vi "计算结果-快关试验.vi"(3 "试验模式":string="快关L1", 5 "油动机试验路径":path=path "D:/研究生/课程/油动机项目/实验文件夹/195-15-6203-018/GV1") -> (0 "计算参数 out":T1, 1 "输入参数":T2, 2 "快关实验":cluster{dbl, "Sampling Rate":dbl, dbl[][]}(graph) caption="当前试验模式：快关试验L1")   [LabVIEW 2013]
uses:
  <vilib>/Analysis/3filter.llb/Filter Passband Type.ctl
  <vilib>/Utility/config.llb/Read Key (String).vi
  <vilib>/Analysis/3filter.llb/Butterworth Filter (DBL).vi
  <vilib>/Analysis/NI_AALBase.lvlib
  <vilib>/Utility/config.llb/NI_LVConfig.lvlib
panel:
  in  "计算参数":T1
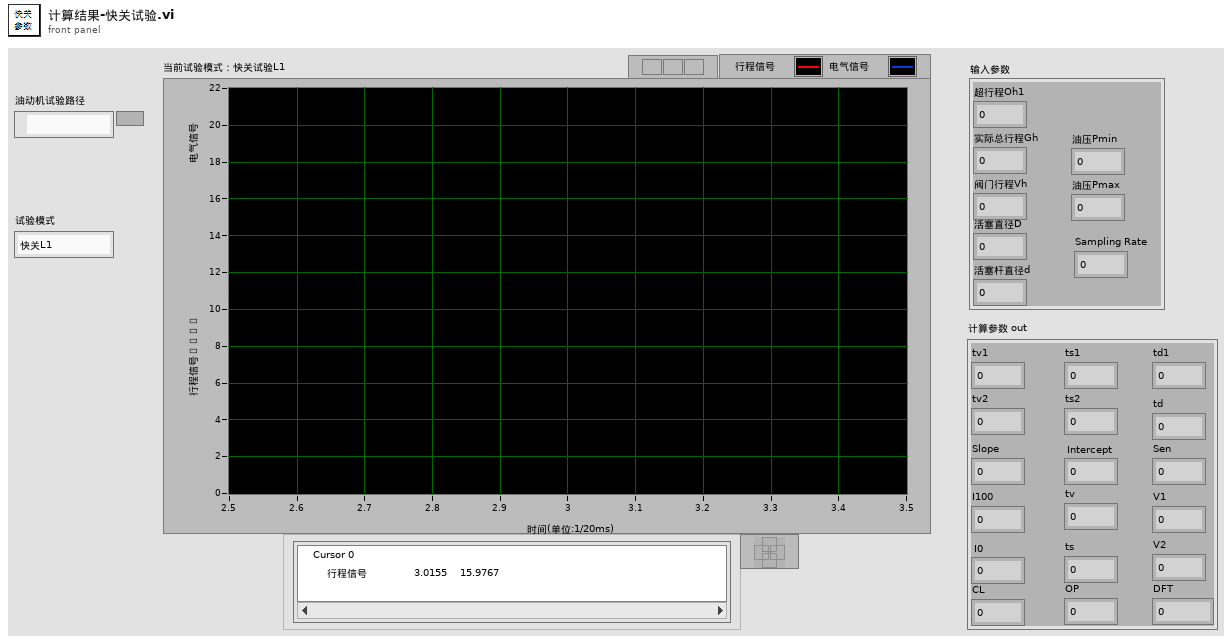
[diagram p1: front panel]
types:
  T1 = cluster{"tv1":dbl, "tv2":dbl, "tv":dbl, "ts1":dbl, "ts2":dbl, "ts":dbl, "td1":dbl, "td":dbl, "Slope":dbl, "Intercept":dbl, "I100":dbl, "I0":dbl, "Sen":dbl, "V1":dbl, "V2":dbl, "CL":dbl, "OP":dbl, "DFT":dbl}
  T2 = cluster{"超行程Oh1":dbl, "实际总行程Gh":dbl, "阀门行程Vh":dbl, "活塞直径D":dbl, "活塞杆直径d":dbl, "油压Pmin":dbl, "油压Pmax":dbl, "Sampling Rate":dbl}
  T3 = typedef "NI_AALBase.lvlib/Filter Passband Type.ctl" = enum32{"Lowpass", "Highpass", "Bandpass", "Bandstop"}
  T4 = enum16{"open", "open or create", "create or replace", "create", "open (read-only)"}
  T5 = typedef "NI_LVConfig.lvlib/Config Data RefNum.ctl" = refnum<k1>
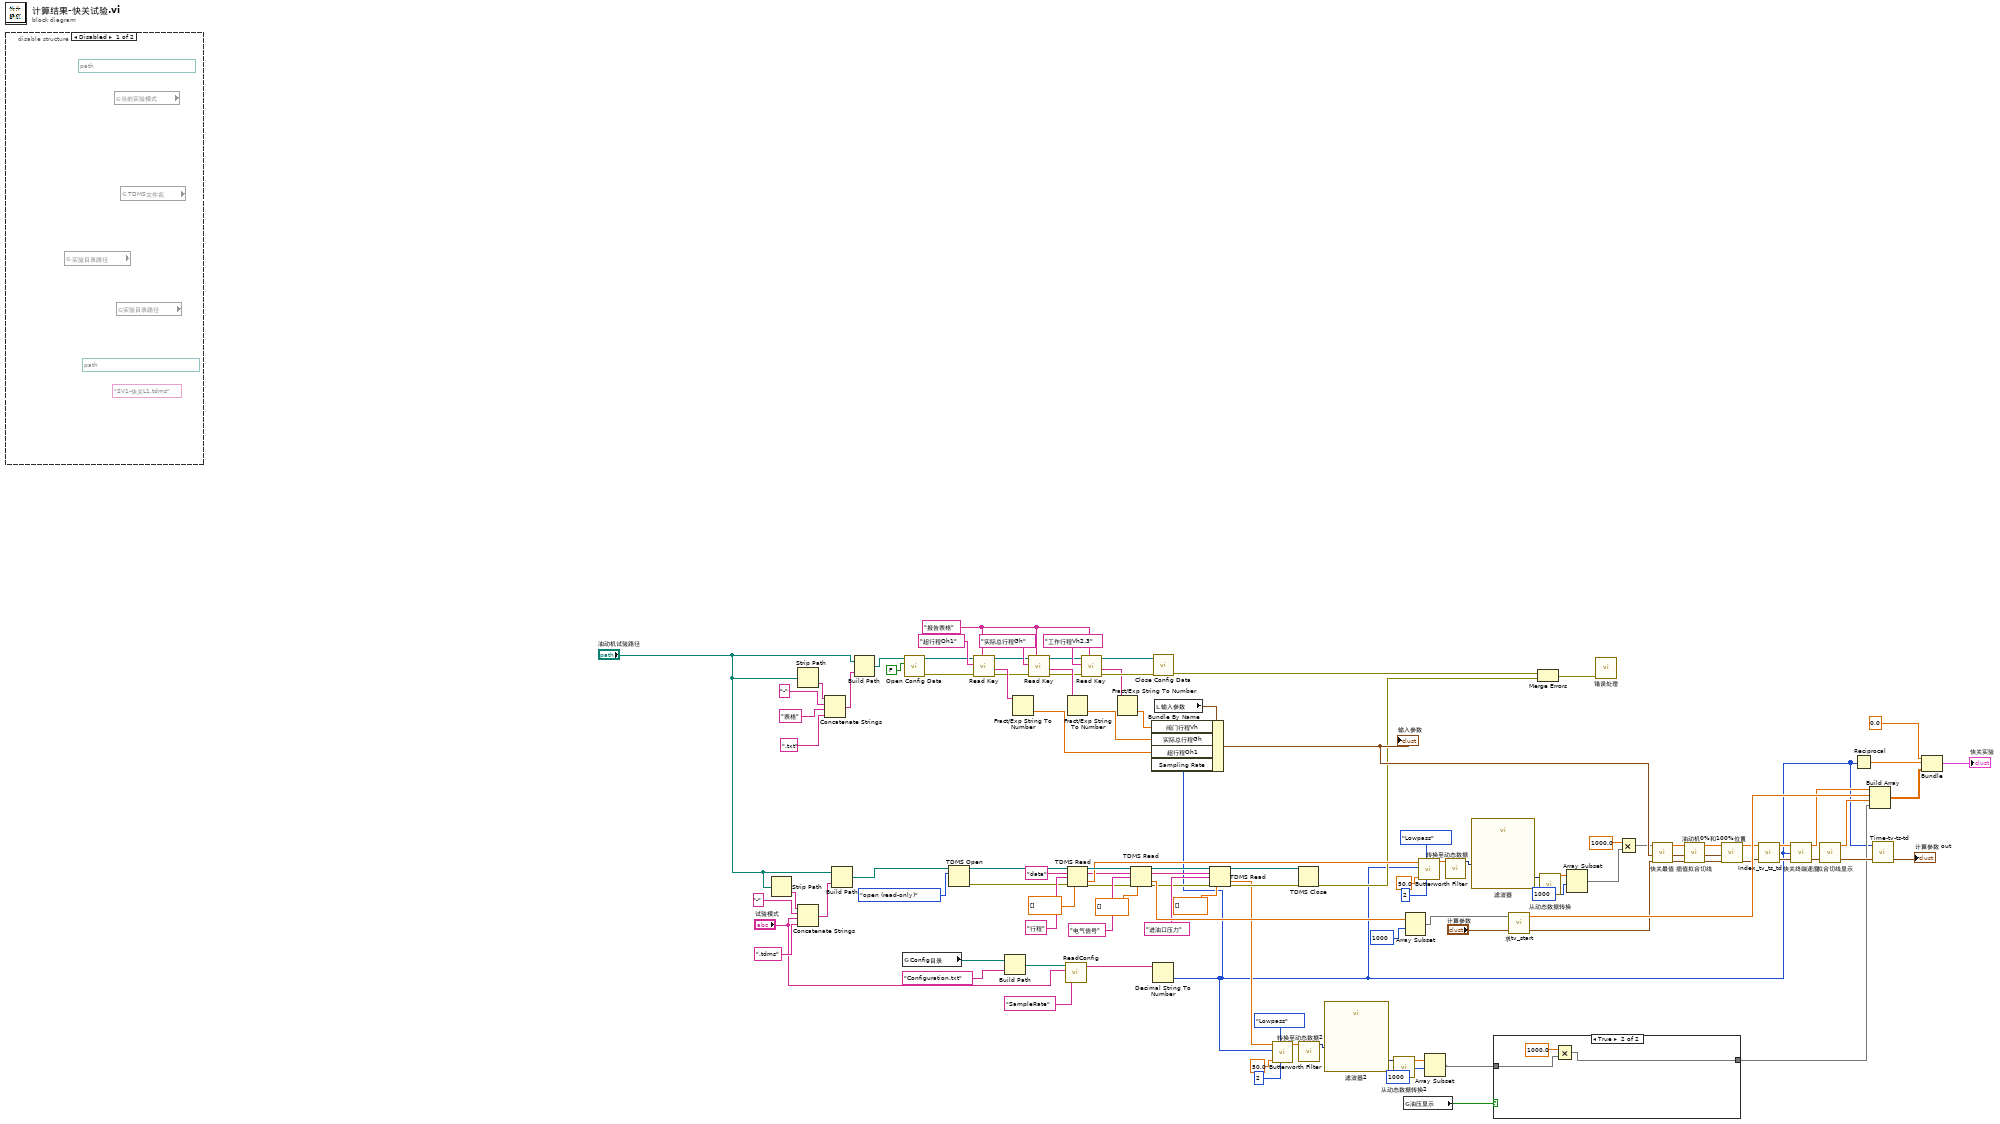
[diagram p0: block diagram]
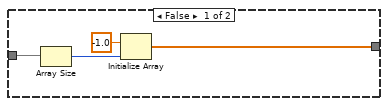
[diagram p2: hidden frame]
diagram:
  w73 = "报告表格" ("section")
  n1 = disable-structure shown="Disabled" {
    frame Disabled {
      (unwired) "SV1-快关L1.tdms"
      (unwired) path "C:/Users/Xiang MU/Desktop/实验文件夹/DR96-03-5/SV1"
      (unwired) path "C:/Users/Xiang MU/Desktop/实验文件夹/DR96-03-5/SV1/SV1-表格.txt"
      n2 = global read "实验目录路径.vi" "实验目录路径"() -> ()  [unwired: 1 out]
      n3 = global read "当前实验模式.vi" "当前实验模式"() -> ()  [unwired: 1 out]
      n4 = global read "实验目录路径.vi" "实验目录路径"() -> ()  [unwired: 1 out]
      n5 = global read "TDMS文件名.vi" "TDMS文件名"() -> ()  [unwired: 1 out]
    }
    frame Enabled {
    }
  }
  n6 = Strip Path(path="油动机试验路径") -> (name=w54:string)  [unwired: 1 out]
  n7 = Strip Path(path="油动机试验路径") -> (name=w49:string)  [unwired: 1 out]
  n8 = Concatenate Strings(w54, "-" ("string"), "试验模式", ".tdms") -> (w53:string)
  n9 = Concatenate Strings(w49, "-" ("string"), "表格" ("string"), ".txt") -> (w45:string)
  n10 = Build Path(base path="油动机试验路径", name or relative path=w53) -> (appended path=w52:path)
  n11 = Build Path(base path="油动机试验路径", name or relative path=w45) -> (appended path=w43:path)
  n12 = global read "Config目录.vi" "Config目录"() -> (w28:path)
  n13 = call <vilib>:"Open Config Data.vi"("create file if necessary (T)"=FALSE, "configuration file path"=w43) -> ("error out"=w58:errorcluster, "refnum"=w57:T5)  [unwired: 7 in, 1 out]
  n14 = TDMS Open(10:T4."open (read-only)" ("operation (0:open)"), 11:w52) -> (0:w26:errorcluster, 3:w55:refnum<k34>)  [unwired: 5 in]
  n15 = call-poly <vilib>:"Read Key.vi"("section"=w73, "error in (no error)"=w58, "key"="超行程Oh1", "refnum"=w57) -> ("error out"=w69:errorcluster, "value"=w76:string, "refnum out"=w70:T5)  [unwired: 4 in, 1 out]
  n16 = Build Path(base path=w28, name or relative path="Configuration.txt") -> (appended path=w27:path)
  n17 = Fract/Exp String To Number(string=w76) -> (number=w90:dbl)  [unwired: 3 in, 1 out]
  n18 = call-poly <vilib>:"Read Key.vi"("section"=w73, "error in (no error)"=w69, "key"="实际总行程Gh" ("default value"), "refnum"=w70) -> ("error out"=w71:errorcluster, "value"=w77:string, "refnum out"=w72:T5)  [unwired: 4 in, 1 out]
  n19 = call "ReadConfig.vi"("Key"="SampleRate", "Section"="试验模式", "Path"=w27) -> ("Value"=w32:string)  [unwired: 1 in, 2 out]
  n20 = Fract/Exp String To Number(string=w77) -> (number=w89:dbl)  [unwired: 3 in, 1 out]
  n21 = TDMS Read(0:w55, 5:"data" ("组名称输入"), 7:"行程" ("组名称输入"), 11:w26, 12:dbl[] []) -> (4:w86:refnum<k34>, 6:w15:string, 10:w81:dbl[], 15:w25:errorcluster)  [unwired: 3 in, 2 out]
  n22 = call-poly <vilib>:"Read Key.vi"("section"=w73, "error in (no error)"=w71, "key"="工作行程Vh2.3", "refnum"=w72) -> ("error out"=w79:errorcluster, "value"=w78:string, "refnum out"=w80:T5)  [unwired: 4 in, 1 out]
  n23 = Fract/Exp String To Number(string=w78) -> (number=w88:dbl)  [unwired: 3 in, 1 out]
  n24 = TDMS Read(0:w86, 5:w15, 7:"电气信号" ("组名称输入"), 11:w25, 12:dbl[] []) -> (4:w19:refnum<k34>, 6:w14:string, 10:w98:dbl[], 15:w16:errorcluster)  [unwired: 3 in, 2 out]
  n25 = Decimal String To Number(string=w32) -> (number=w1:i32)  [unwired: 2 in, 1 out]
  n26 = call <vilib>:"Close Config Data.vi"("error in (no error)"=w79, "refnum"=w80) -> ("error out"=w24:errorcluster)  [unwired: 8 in, 1 out]
  n27 = local read "输入参数"() -> (w91:T2)
  n28 = Bundle By Name(cluster=w91, "阀门行程Vh"=w88, "实际总行程Gh"=w89, "超行程Oh1"=w90, "Sampling Rate"=w1) -> (w103:T2)
  "输入参数" <- w103
  n29 = TDMS Read(0:w19, 5:w14, 7:"进油口压力" ("组名称输入"), 11:w16, 12:dbl[] []) -> (4:w18:refnum<k34>, 10:w2:dbl[], 15:w17:errorcluster)  [unwired: 3 in, 3 out]
  n30 = call-poly <vilib>:"Butterworth Filter.vi"("order"=2, "filter type"=Filter_Passband_Type."Lowpass", "low cutoff freq: fl"=50.0, "sampling freq: fs"=w1, "X"=w2) -> ("Filtered X"=w7:dbl[])  [unwired: 3 in, 1 out]
  n31 = TDMS Close(8:w17, 11:w18) -> (0:w23:errorcluster)  [unwired: 1 out]
  n32 = call "转换至动态数据2"("Array"=w7) -> ("Dynamic Data Type"=w8:dynamicdata)  [unwired: 3 in]
  n33 = call "滤波器2"("Signal"=w8) -> ("Filtered Signal"=w9:dynamicdata)  [unwired: 9 in, 1 out]
  n34 = call "从动态数据转换2"("Dynamic Data Type"=w9) -> ("Array"=w10:dbl[])  [unwired: 3 in]
  n35 = global read "油压显示.vi" "油压显示"() -> (w13:bool)
  n36 = Array Subset(array=w98, index=1000) -> (w100:dbl[])  [unwired: 1 in]
  n37 = call-poly <vilib>:"Butterworth Filter.vi"("order"=2, "filter type"=Filter_Passband_Type."Lowpass", "low cutoff freq: fl"=50.0, "sampling freq: fs"=w1, "X"=w81) -> ("Filtered X"=w65:dbl[])  [unwired: 3 in, 1 out]
  n38 = Array Subset(array=w10, index=1000) -> (w3:dbl[])  [unwired: 1 in]
  n39 = call "转换至动态数据"("Array"=w65) -> ("Dynamic Data Type"=w66:dynamicdata)  [unwired: 3 in]
  n40 = call "滤波器"("Signal"=w66) -> ("Filtered Signal"=w67:dynamicdata)  [unwired: 9 in, 1 out]
  n41 = case shown="True" w13 {
    tunnel: w3 -> [w114 w116]
    tunnel: [w111 w115] -> w12
    frame False {
      n42 = Array Size(array=w114) -> (size(s)=w113:i32)
      n43 = Initialize Array(-1.0 ("element"), w113) -> (w111:dbl[])
    }
    frame True {
      n44 = Multiply(x=1000.0 ("low cutoff freq: fl"), y=w116) -> (x*y=w115:dbl[])
    }
  }
  n45 = call "求tv_start.vi"("计算参数 in"="计算参数", "Array in"=w100) -> ("计算参数 out"=w95:T1, "Array out"=w109:dbl[])  [unwired: 2 in]
  n46 = Merge Errors(w24, w23) -> (w22:errorcluster)
  n47 = call "从动态数据转换"("Dynamic Data Type"=w67) -> ("Array"=w96:dbl[])  [unwired: 3 in]
  n48 = Array Subset(array=w96, index=1000) -> (w101:dbl[])  [unwired: 1 in]
  n49 = call "错误处理.vi"("error in (no error)"=w22) -> ()  [unwired: 2 in]
  n50 = Multiply(x=1000.0 ("low cutoff freq: fl"), y=w101) -> (x*y=w82:dbl[])
  n51 = call "快关最值.vi"("计算参数 in"=w95, "输入参数 in"=w103, "Array in"=w82) -> ("计算参数 out"=w92:T1, "输入参数 out"=w104:T2, "Array out"=w83:dbl[])  [unwired: 2 in]
  n52 = call "插值拟合切线.vi"("计算参数 in"=w92, "输入参数 in"=w104, "Array in"=w83) -> ("计算参数 out"=w93:T1, "输入参数 out"=w105:T2, "Array out"=w106:dbl[])  [unwired: 2 in]
  n53 = call "油动机0%和100%位置.vi"("计算参数 in"=w93, "输入参数 in"=w105, "Array in"=w106) -> ("计算参数 out"=w94:T1, "Array out"=w107:dbl[])  [unwired: 2 in, 1 out]
  n54 = call "Index_tv_ts_td.vi"("计算参数 in"=w94, "Array in"=w107) -> ("计算参数 out"=w36:T1, "Array out"=w34:dbl[])  [unwired: 2 in]
  n55 = call "快关终端速度.vi"("计算参数 in"=w36, "Sampling Rate"=w1, "Array in"=w34) -> ("计算参数 out"=w35:T1, "Array out"=w33:dbl[])  [unwired: 1 in]
  n56 = call "拟合切线显示.vi"("计算参数 in"=w35) -> ("计算参数 out"=w38:T1, "Array out"=w108:dbl[])  [unwired: 3 in]
  n57 = Reciprocal(x=w1) -> (1/x=w39:dbl)
  n58 = Build Array(w33, w109, w108, w12) -> (w41:dbl[][])
  n59 = call "Time-tv-ts-td.vi"("计算参数 in"=w38, "SamplingRate"=w1) -> ("计算参数 out"=→"计算参数 out":T1)  [unwired: 3 in]
  n60 = Bundle(0.0, w39, w41) -> (→"快关实验":cluster{dbl, dbl, dbl[][]})  [unwired: 1 in]
